vi "genIOL_Injection3.vi"(4 "Initial guess":dbl[](array[numeric])=[-67.99974822998047, 12.682350158691406, -0.8997803330421448, -0.012297453358769417], 5 "True_endPt":dbl[](array[numeric])=[8.48840241312517, 12.608494085712664, 1.4642729158965477], 6 "DH Params":cluster{"d_DH":dbl[][], "ty":dbl[][]}, 7 "endJ5":dbl=3200.0, 8 "OCT offset":dbl=11.0, 9 "endPt":dbl[](array[numeric])=[8.48840241312517, 12.608494085712664, 1.4642729158965477], 10 "PC path":path=path "D:/IRISSoft LV2016 beta/Host Demo/ThorlabsData/Eye1/VSCAN_0008.raw", 11 "Iris path":path=path "D:/IRISSoft LV2016 beta/Host Demo/ThorlabsData/Eye1/VSCAN_0007.raw") -> (0 "Whole_traj":dbl[][](array[numeric]), 1 "Inject_traj":dbl[][](array[numeric]))   [LabVIEW 2016]
uses:
  <vilib>/Math Plots/3D Math Plots/3D Scatter/3D Scatter XCtrl/3D Scatter.xctl
  <vilib>/Utility/file.llb/Read Delimited Spreadsheet (DBL).vi
  <vilib>/Utility/file.llb/Write Delimited Spreadsheet (DBL).vi
  <vilib>/Math Plots/3D Math Plots/3D Scatter/3D Scatter Datatype/Public/Plot Helper (Vector).vi
  <vilib>/Analysis/NI_AALBase.lvlib
  <vilib>/Analysis/1siggen.llb/Ramp Pattern by Samples.vi
  <vilib>/gmath/NI_Gmath.lvlib
  Subsystems/Global Variables.vi
  <vilib>/Math Plots/3D Math Plots/3D Scatter/3D Scatter Datatype/3D Scatter Datatype.lvclass
  <vilib>/Math Plots/3D Math Plots/3D Plot/3D Plot Datatype/3D Plot Datatype.lvclass
panel:
  out "Implement joint angles":dbl[][](array[numeric])
  in  "Theta":dbl
  out "Actual Injection Plot 2":refnum<class "3D Plot Datatype.lvclass">[](xcontrol)
  out "current loop # 2":dbl
  out "Actual joint angles":dbl[][](array[numeric])
  out "Planned joint angles":dbl[][](array[numeric])
  out "Planned injection":dbl[][](array[numeric])
  out "time":dbl[](array[numeric])
  out "Implement joint angles":dbl[][](graph)
  out "min dist":dbl
  out "Planed joint angles":dbl[][](graph)
  out "Actual joint angles":dbl[][](graph)
  out "traj":dbl[][](array[numeric])
  out "max dist":dbl
  out "Offset":dbl[][](array[numeric])
  out "Planed Injection Plot":refnum<class "3D Plot Datatype.lvclass">[](xcontrol)
  out "current loop #":dbl
  out "x coordinates size 3":dbl
  out "x coordinates size 2":dbl
  out "x coordinates size":dbl
  out "x coordinates":dbl[](array[numeric])
  out "z coordinates":dbl[](array[numeric]) format="%#_13g"
  out "y coordinates":dbl[](array[numeric]) format="%#_13g"
  out "x coodi 2nd":dbl[](array[numeric]) format="%#_13g"
  in  "Total Time":dbl=60.0
  in  "Arm ID Ind":i32
  in  "Tip out Posit":dbl[](array[numeric])=[0.0, 0.0, 0.0] caption="Position [mm]" format="%#.3f"
  out "zVisTraj":dbl[](array[numeric]) format="%_6g"
  out "yVisTraj":dbl[](array[numeric]) format="%_6g"
  out "xVisTraj":dbl[](array[numeric]) format="%_6g"
  in  "Sampling Rate [Hz]":i32=1000
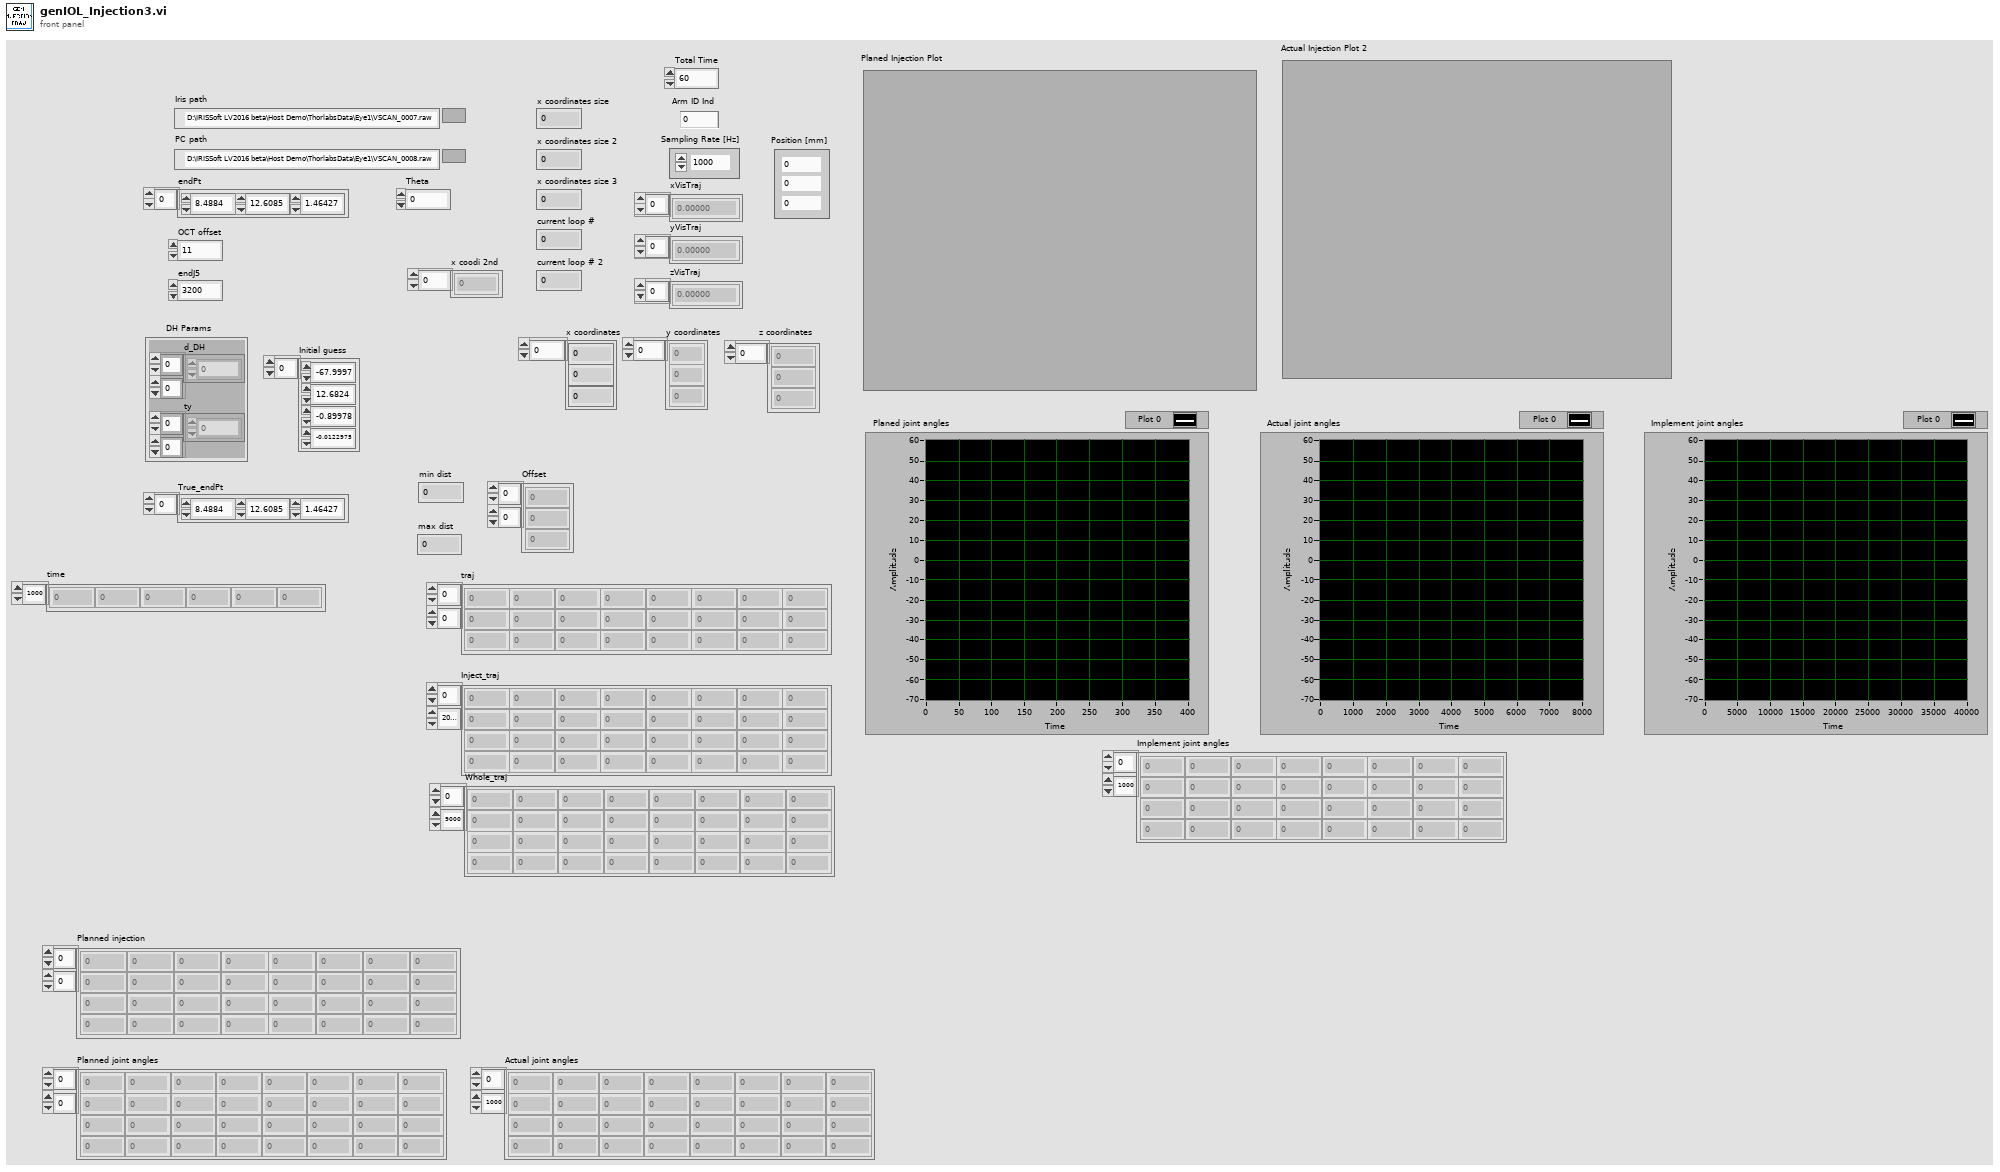
[diagram p1: front panel]
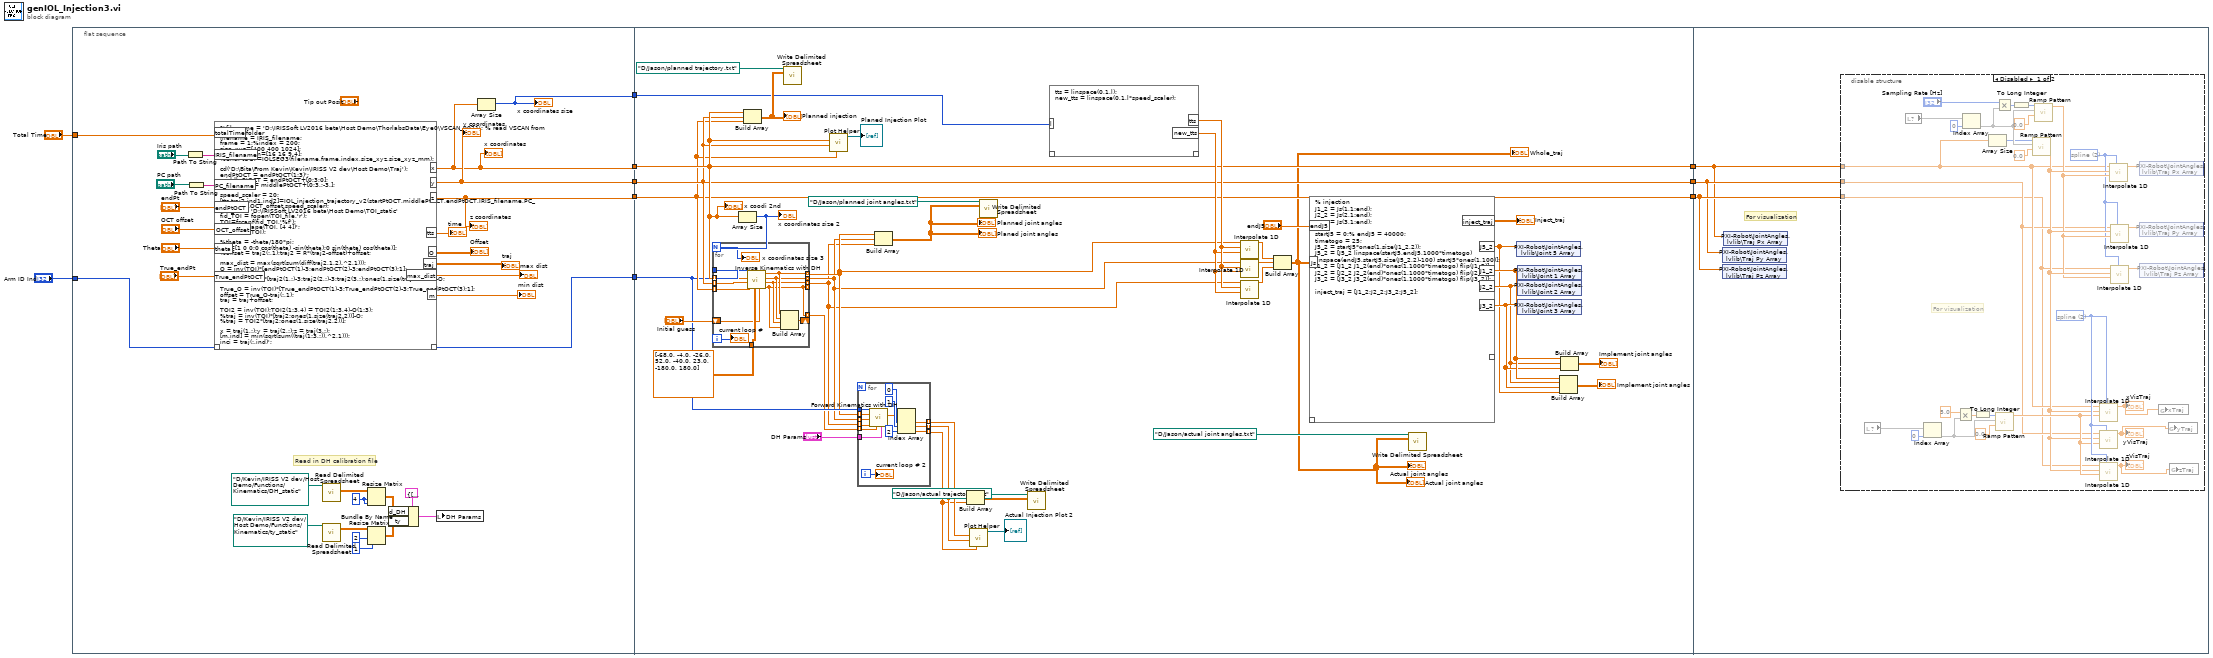
[diagram p0: block diagram]
diagram:
  n1 = flat-sequence {
    tunnel: "Arm ID Ind" -> [w13]
    tunnel: [w37] -> w6
    tunnel: [w39] -> w5
    tunnel: [w38] -> w4
    tunnel: "Total Time" -> [w40]
    tunnel: [w25] -> w2
    tunnel: [w13] -> w1
    tunnel: [w68] -> w9
    tunnel: [w67] -> w8
    tunnel: [w66] -> w7
    tunnel: w6 -> [w68]
    tunnel: w5 -> [w67]
    tunnel: w4 -> [w66]
    tunnel: w2 -> [w49]
    tunnel: w1 -> [w60]
    tunnel: w9 -> [w107]
    tunnel: w8 -> [w108]
    tunnel: w7 -> [w109]
    frame #0 {
      w22 = 4 ("number of rows")
      # "Read in DH calibration file"
      n2 = Path To String(path="Iris path") -> (string=w32:string)
      n3 = Path To String(path="PC path") -> (string=w33:string)
      n4 = script code="%filename = 'D:\\IRISSoft LV2016 beta\\Host Demo\\ThorlabsData\\Eye0\\VSCAN_0021'; % read VSCAN from network folder \nfilename = IRIS_filename;\nframe = 1;%index = 200;\nsize_xyz=[400 400 1024];\nsize_xyz_mm=[16 16 9.4];\n%endPtOCT=IOLSEG3(filename,frame,index,size_xyz,size_xyz_mm);\n\ncd('D:\\Bita\\From Kevin\\Kevin\\IRISS V2 dev\\Host Demo\\Traj');\nendPtOCT = endPtOCT(1:3)';\nmiddlePtOCT = endPtOCT+[0;3;0];\nstartPtOCT = middlePtOCT+[0;3.;-3.];\n\nspeed_scaler = 20;\n[tts,traj2,ind1,ind2]=IOL_injection_trajectory_v2(startPtOCT,middlePtOCT,endPtOCT,IRIS_filename,PC_filename,OCT_offset,speed_scaler);\nTOI_file= 'D:\\IRISSoft LV2016 beta\\Host Demo\\TOI_static'\nfid_TOI = fopen(TOI_file,'r');\nTOI=fscanf(fid_TOI,'%f');\nTOI= reshape(TOI, [4 4])';\nfclose(fid_TOI);\n\n%theta = -theta/180*pi;\n%R=[1 0 0;0 cos(theta) -sin(theta);0 sin(theta) cos(theta)];\n%offset = traj2(:,1);traj2 = R*(traj2-offset)+offset;\n\nmax_dist = max(sqrt(sum(diff(traj2,1,2).^2,1)));\nO = inv(TOI)*[endPtOCT(1)-3;endPtOCT(2)-3;endPtOCT(3);1];\n\ntraj = inv(TOI)*[traj2(1,:)-3;traj2(2,:)-3;traj2(3,:);ones(1,size(traj2,2))];%-O;\n\nTrue_O = inv(TOI)*[True_endPtOCT(1)-3;True_endPtOCT(2)-3;True_endPtOCT(3);1];\noffset = True_O-traj(:,1);\ntraj = traj+offset;\n\nTOI2 = inv(TOI);TOI2(1:3,4) = TOI2(1:3,4)-O(1:3);\n%traj = inv(TOI)*[traj2;ones(1,size(traj2,2))]-O;\n%traj = TOI2*[traj2;ones(1,size(traj2,2))];\n\nx = traj(1,:);y = traj(2,:);z = traj(3,:);\n[m,ind] = min(sqrt(sum((traj(1:3,:)).^2,1)));\ninci = traj(:,ind)';"("totalTime"=w40, "IRIS_filename"=w32, "PC_filename"=w33, "endPtOCT"="endPt", "OCT_offset"="OCT offset", "theta"="Theta", "True_endPtOCT"="True_endPt") -> ("x"=w37:dbl[], "y"=w39:dbl[], "z"=w38:dbl[], "O"=→"Offset":dbl[][], "max_dist"=→"max dist":dbl, "traj"=→"traj":dbl[][], "m"=→"min dist":dbl, "tts"=→"time":dbl[])  [unwired: 1 in, 1 out]
      "y coordinates" <- w39
      "z coordinates" <- w38
      "x coordinates" <- w37
      n5 = call-poly <vilib>:"Read Delimited Spreadsheet.vi"("file path (dialog if empty)"=path "D:/Kevin/IRISS V2 dev/Host Demo/Functions/Kinematics/DH_static" ("file path (use dialog)")) -> ("all rows"=w23:dbl[][])  [unwired: 9 in, 5 out]
      n6 = call-poly <vilib>:"Read Delimited Spreadsheet.vi"("file path (dialog if empty)"=path "D:/Kevin/IRISS V2 dev/Host Demo/Functions/Kinematics/ty_static" ("file path (use dialog)")) -> ("all rows"=w21:dbl[][])  [unwired: 9 in, 5 out]
      n7 = Resize Matrix(1:w22, 2:w22, 4:w23) -> (0:w17:dbl[][])
      n8 = Resize Matrix(1:1 ("number of columns"), 2:2 ("number of rows"), 4:w21) -> (0:w16:dbl[][])
      n9 = Bundle By Name(cluster=cluster{"d_DH":dbl[][], "ty":dbl[][]} {"d_DH"=[[0.0, -0.04858099004841317, 1.1971672750675049, 0.0], [0.0, -1.576475511297109, 0.0, 0.0], [-0.3552491783526254, 0.0, -1.1064589410656984, 0.2058446720735121], [-1.0573457532495087, 1.0278049025155533, 0.011917110633363169, -0.004023577880993236]], "ty"=[[0.04320445582455471], [0.011728642746432275]]} ("input cluster"), "d_DH"=w17, "ty"=w16) -> (w14:cluster{"d_DH":dbl[][], "ty":dbl[][]})
      n10 = local write "DH Params"(w14) -> ()
      n11 = Array Size(array=w37) -> (size(s)=w25:i32)
      "x coordinates size" <- w25
    }
    frame #1 {
      n12 = Array Size(array=w68) -> (size(s)=w79:i32)
      "x coordinates size 2" <- w79
      n13 = for {
        N: w79 -> [w106]
        tunnel: w60 -> [w103]
        tunnel: w68 -> [w102] mode=indexing
        tunnel: w67 -> [w101] mode=indexing
        tunnel: w66 -> [w100] mode=indexing
        tunnel: [w96] -> w53 mode=indexing
        tunnel: [w97] -> w54 mode=indexing
        tunnel: [w95] -> w52 mode=indexing
        tunnel: dbl[][] [[-68.0, -4.0], [-26.0, 52.0], [-40.0, 23.0], [-180.0, 180.0]] ("Joint Limits") -> [w99]
        shift-right: [w104] -> _
        shift-left: "Initial guess" -> [w98]
        tunnel: [w94] -> _ mode=indexing
        tunnel: [w94] -> w46 mode=indexing
        i -> [w105]
        n14 = call "Inverse Kinematics with DH.vi"("Initial guess"=w98, "Joint Limits"=w99, "armID"=w103, "z"=w100, "y"=w101, "x"=w102) -> ("j4"=w94:dbl, "j3"=w95:dbl, "j2"=w96:dbl, "j1"=w97:dbl)  [unwired: 2 in]
        n15 = Build Array(w97, w96, w95, w94) -> (w104:dbl[])
        "x coordinates size 3" <- w106
        "current loop #" <- w105
      }
      n16 = Build Array(w68, w67, w66) -> (w65:dbl[][])
      "Planned injection" <- w65
      n17 = call-poly <vilib>:"Write Delimited Spreadsheet.vi"("file path (dialog if empty)"=path "D:/Jason/planned trajectory.txt", "2D data"=w65) -> ()  [unwired: 12 in, 2 out]
      n18 = call-poly <vilib>:"Plot Helper.vi"("z vector"=w66, "y vector"=w67, "x vector"=w68) -> ("3D Plot lvclass Array out"=→"Planed Injection Plot":refnum<class "3D Plot Datatype.lvclass">[])  [unwired: 3 in, 5 out]
      n19 = for {
        tunnel: w60 -> [w86]
        tunnel: w54 -> [w87] mode=indexing
        tunnel: w53 -> [w85] mode=indexing
        tunnel: w52 -> [w84] mode=indexing
        tunnel: [w90] -> w59 mode=indexing
        tunnel: [w89] -> w58 mode=indexing
        tunnel: [w88] -> w57 mode=indexing
        tunnel: "DH Params" -> [w82]
        tunnel: w46 -> [w80] mode=indexing
        i -> [w81]
        n20 = call "Forward Kinematics with DH.vi"("DH Params"=w82, "j4"=w80, "j3"=w84, "j2"=w85, "j1"=w87, "armID"=w86) -> ("XYZ With DH Calibration"=w83:dbl[])  [unwired: 3 in, 2 out]
        n21 = Index Array(array=w83, index #1=0 ("index"), index #2=1 ("index"), index #3=2 ("index")) -> (element #1=w90:dbl, element #2=w89:dbl, element #3=w88:dbl)
        "current loop # 2" <- w81
      }
      n22 = Build Array(w54, w53, w52) -> (w63:dbl[][])
      "Planed joint angles" <- w63
      "Planned joint angles" <- w63
      n23 = Build Array(w59, w58, w57) -> (w56:dbl[][])
      n24 = call-poly <vilib>:"Plot Helper.vi"("z vector"=w57, "y vector"=w58, "x vector"=w59) -> ("3D Plot lvclass Array out"=→"Actual Injection Plot 2":refnum<class "3D Plot Datatype.lvclass">[])  [unwired: 3 in, 5 out]
      n25 = call-poly <vilib>:"Write Delimited Spreadsheet.vi"("file path (dialog if empty)"=path "D:/Jason/planned joint angles.txt", "2D data"=w63) -> ()  [unwired: 12 in, 2 out]
      n26 = call-poly <vilib>:"Write Delimited Spreadsheet.vi"("file path (dialog if empty)"=path "D:/Jason/actual trajectory2.txt", "2D data"=w56) -> ()  [unwired: 12 in, 2 out]
      n27 = script code="tts = linspace(0,1,l);\nnew_tts = linspace(0,1,l*speed_scaler);"("l"=w49) -> ("new_tts"=w75:dbl[], "tts"=w76:dbl[])  [unwired: 1 in, 1 out]
      n28 = call <vilib>:"Interpolate 1D.vi"("xi"=w75, "X"=w76, "Y"=w54) -> ("yi"=w74:dbl[])  [unwired: 6 in, 2 out]
      n29 = call <vilib>:"Interpolate 1D.vi"("xi"=w75, "X"=w76, "Y"=w53) -> ("yi"=w73:dbl[])  [unwired: 6 in, 2 out]
      n30 = call <vilib>:"Interpolate 1D.vi"("xi"=w75, "X"=w76, "Y"=w52) -> ("yi"=w72:dbl[])  [unwired: 6 in, 2 out]
      n31 = Build Array(w74, w73, w72) -> (w48:dbl[][])
      "Actual joint angles" <- w48
      "Whole_traj" <- w48
      "Actual joint angles" <- w48
      n32 = script code="% injection\nJ1_2 = Js(1,1:end);\nJ2_2 = Js(2,1:end);\nJ3_2 = Js(3,1:end);\n\nstartJ5 = 0;% endJ5 = 40000;\ntimetogo = 25;\nJ5_2 = startJ5*ones(1,size(J1_2,2));\nJ5_2 = [J5_2 linspace(startJ5,endJ5,1000*timetogo) linspace(endJ5,startJ5,size(J5_2,2)-100) startJ5*ones(1,100)];\nJ1_2 = [J1_2 J1_2(end)*ones(1,1000*timetogo) flip(J1_2)];\nJ2_2 = [J2_2 J2_2(end)*ones(1,1000*timetogo) flip(J2_2)];\nJ3_2 = [J3_2 J3_2(end)*ones(1,1000*timetogo) flip(J3_2)];\n\ninject_traj = [J1_2;J2_2;J3_2;J5_2];"("Js"=w48, "endJ5"="endJ5") -> ("J1_2"=w45:dbl[], "J2_2"=w43:dbl[], "J3_2"=w44:dbl[], "J5_2"=w42:dbl[], "inject_traj"=→"Inject_traj":dbl[][])  [unwired: 1 in, 1 out]
      n33 = call-poly <vilib>:"Write Delimited Spreadsheet.vi"("file path (dialog if empty)"=path "D:/Jason/actual joint angles.txt", "2D data"=w48) -> ()  [unwired: 12 in, 2 out]
      n34 = shared-variable "PXI-Robot\\JointAngles.lvlib\\Joint 5 Array"(w42) -> ()  [unwired: 1 in, 1 out]
      n35 = shared-variable "PXI-Robot\\JointAngles.lvlib\\Joint 1 Array"(w45) -> ()  [unwired: 1 in, 1 out]
      n36 = shared-variable "PXI-Robot\\JointAngles.lvlib\\Joint 2 Array"(w43) -> ()  [unwired: 1 in, 1 out]
      n37 = shared-variable "PXI-Robot\\JointAngles.lvlib\\Joint 3 Array"(w44) -> ()  [unwired: 1 in, 1 out]
      n38 = Build Array(w45, w43, w44, w42) -> (→"Implement joint angles":dbl[][])
      n39 = Build Array(w45, w43, w44) -> (→"Implement joint angles":dbl[][])
      "x coodi 2nd" <- w68
    }
    frame #2 {
      # "For visualization"
      n40 = shared-variable "PXI-Robot\\JointAngles.lvlib\\Traj Py Array"(w108) -> ()  [unwired: 1 in, 1 out]
      n41 = shared-variable "PXI-Robot\\JointAngles.lvlib\\Traj Pz Array"(w109) -> ()  [unwired: 1 in, 1 out]
      n42 = shared-variable "PXI-Robot\\JointAngles.lvlib\\Traj Px Array"(w107) -> ()  [unwired: 1 in, 1 out]
      n43 = disable-structure shown="Disabled" {
        disable-tunnel: w107 -> [w115 _]
        disable-tunnel: w108 -> [w114 _]
        disable-tunnel: w109 -> [w113 _]
        frame Disabled {
          w127 = 2 items=["nearest", "linear", "spline", "cubic Hermite", "Lagrange"] ("method")
          w116 = 2 items=["nearest", "linear", "spline", "cubic Hermite", "Lagrange"] ("method")
          # "For visualization"
          n44 = local read item#-1() -> (w121)
          n45 = local read item#-1() -> (w139)
          n46 = Index Array(array=w121, index=0) -> (element=w122)
          n47 = Multiply(x=5.0, y=w122) -> (x*y=w124:dbl)
          n48 = Index Array(array=w139, index=0) -> (element=w132)
          n49 = To Long Integer(number=w124) -> (32bit integer=w125:i32)
          n50 = Array Size(array=w115) -> (size(s)=w131:i32)
          n51 = call-poly <vilib>:"Ramp Pattern.vi"("start"=0.0, "end"=w122, "samples"=w125) -> ("Ramp Pattern"=w119:dbl[])  [unwired: 7 in, 1 out]
          n52 = Multiply(x="Sampling Rate [Hz]", y=w132) -> (x*y=w135:i32)
          n53 = To Long Integer(number=w135) -> (32bit integer=w136:i32)
          n54 = call-poly <vilib>:"Ramp Pattern.vi"("start"=0.0, "end"=w132, "samples"=w131) -> ("Ramp Pattern"=w118:dbl[])  [unwired: 7 in, 1 out]
          n55 = call-poly <vilib>:"Ramp Pattern.vi"("start"=0.0, "end"=w132, "samples"=w136) -> ("Ramp Pattern"=w117:dbl[])  [unwired: 7 in, 1 out]
          n56 = call <vilib>:"Interpolate 1D.vi"("method"=w127, "xi"=w119, "X"=w118, "Y"=w115) -> ("yi"=w110:dbl[])  [unwired: 5 in, 2 out]
          "xVisTraj" <- w110
          n57 = call <vilib>:"Interpolate 1D.vi"("method"=w127, "xi"=w119, "X"=w118, "Y"=w114) -> ("yi"=w111:dbl[])  [unwired: 5 in, 2 out]
          "yVisTraj" <- w111
          n58 = call <vilib>:"Interpolate 1D.vi"("method"=w127, "xi"=w119, "X"=w118, "Y"=w113) -> ("yi"=w112:dbl[])  [unwired: 5 in, 2 out]
          "zVisTraj" <- w112
          n59 = call <vilib>:"Interpolate 1D.vi"("method"=w116, "xi"=w117, "X"=w118, "Y"=w115) -> ("yi"=w129:dbl[])  [unwired: 5 in, 2 out]
          n60 = call <vilib>:"Interpolate 1D.vi"("method"=w116, "xi"=w117, "X"=w118, "Y"=w114) -> ("yi"=w130:dbl[])  [unwired: 5 in, 2 out]
          n61 = call <vilib>:"Interpolate 1D.vi"("method"=w116, "xi"=w117, "X"=w118, "Y"=w113) -> ("yi"=w128:dbl[])  [unwired: 5 in, 2 out]
          n62 = shared-variable "PXI-Robot\\JointAngles.lvlib\\Traj Px Array"(w129) -> ()  [unwired: 1 in, 1 out]
          n63 = shared-variable "PXI-Robot\\JointAngles.lvlib\\Traj Py Array"(w130) -> ()  [unwired: 1 in, 1 out]
          n64 = shared-variable "PXI-Robot\\JointAngles.lvlib\\Traj Pz Array"(w128) -> ()  [unwired: 1 in, 1 out]
          n65 = global write "Global Variables.vi" "xTraj"(w110) -> ()
          n66 = global write "Global Variables.vi" "yTraj"(w111) -> ()
          n67 = global write "Global Variables.vi" "zTraj"(w112) -> ()
        }
        frame Enabled {
        }
      }
    }
  }
